vi "Reveal World.vi"(6 "radius":i32 min=0, 8 "y":i32 min=0, 9 "x":i32 min=0, 10 "cost in":dbl[][](array[numeric]), 11 "map reference in":refnum<data-value>) -> (2 "cost out":dbl[][](array[numeric]), 3 "map reference in 2":refnum<data-value>)   [LabVIEW 2013]
uses:
  <vilib>/robotics/Navigation/shared/WorldMap/OccupancyGridWorldMap/NI_Robotics_OccupancyGridWorldMap.lvclass
panel:
  in  "error in (no error)":errorcluster
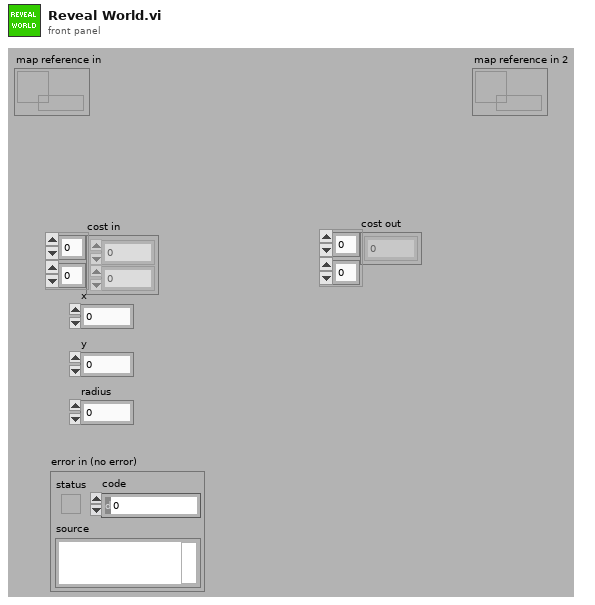
[diagram p1: front panel]
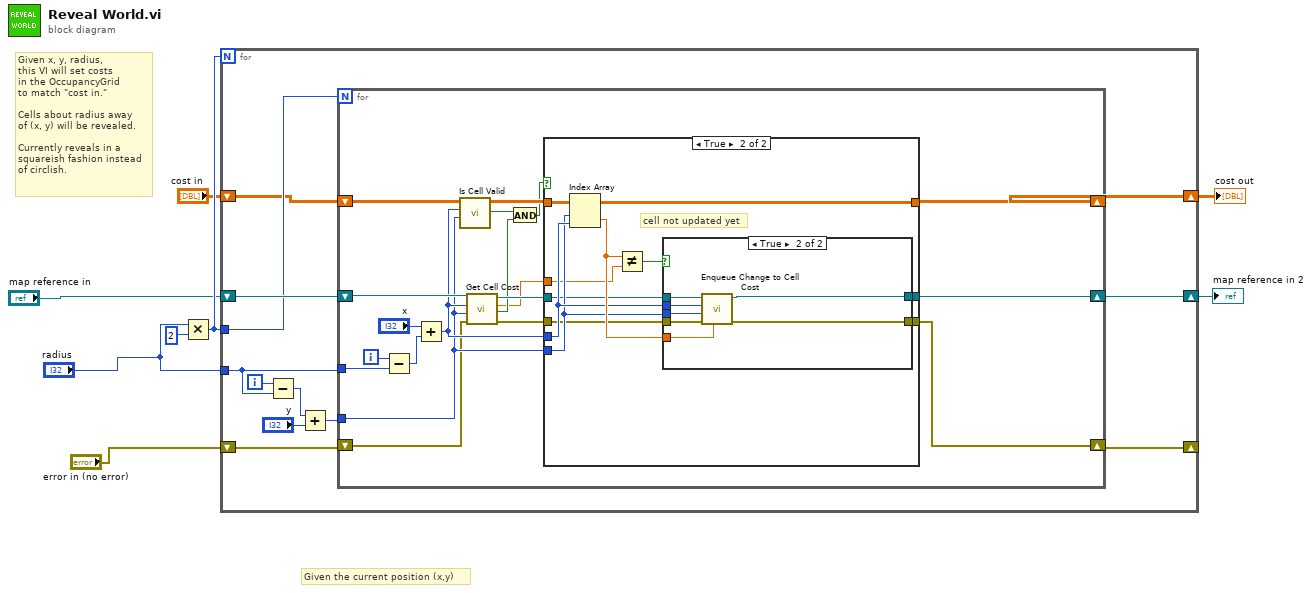
[diagram p0: block diagram]
diagram:
  # "Given the current position (x,y)"
  # "Given x, y, radius,\nthis VI will set costs\nin the OccupancyGrid\nto match \"cost in.\"\n\nCells about radius away\nof (x, y) will be revealed.\n\nCurrently reveals in a \nsquareish fashion instead\nof circlish."
  n1 = Multiply(x="radius", y=2) -> (x*y=w7:i32)
  n2 = for {
    N: w7 -> [_]
    shift-right: [w19] -> w3
    shift-left: "map reference in" -> [w20]
    tunnel: w7 -> [w18]
    tunnel: "radius" -> [w16]
    shift-right: [w14] -> w5
    shift-left: "cost in" -> [w15]
    shift-right: [w9] -> _
    shift-left: "error in (no error)" -> [w10]
    i -> [w17]
    n3 = Subtract(x=w17, y=w16) -> (x-y=w13:i32)
    n4 = Add(x=w13, y="y") -> (x+y=w11:i32)
    n5 = for {
      N: w18 -> [_]
      shift-right: [w21] -> w19
      shift-left: w20 -> [w30]
      tunnel: w16 -> [w38]
      tunnel: w11 -> [w27]
      shift-right: [w35] -> w14
      shift-left: w15 -> [w37]
      shift-right: [w22] -> w9
      shift-left: w10 -> [w24]
      i -> [w39]
      n6 = Subtract(x=w39, y=w38) -> (x-y=w33:i32)
      n7 = Add(x="x", y=w33) -> (x+y=w28:i32)
      n8 = call "Is Cell Valid.vi"("y"=w27, "x"=w28, "cost in"=w37) -> ("Valid"=w31:bool, "cost out"=w36:dbl[][])  [unwired: 7 in]
      n9 = call <vilib>:"Get Cell Cost.vi"("error in (no error)"=w24, "y"=w27, "x"=w28, "map reference in"=w30) -> ("error out"=w23:errorcluster, "found?"=w26:bool, "cost"=w25:dbl, "map reference out"=w29:refnum<data-value>)  [unwired: 4 in]
      n10 = And(x=w31, y=w26) -> (x .and. y?=w34:bool)
      n11 = case shown="True" w34 {
        tunnel: [w42 w52] -> w21
        tunnel: w29 -> [w42 w46]
        tunnel: w28 -> [_ w49]
        tunnel: w27 -> [_ w48]
        tunnel: w36 -> [w41 w43]
        tunnel: [w41 w43] -> w35
        tunnel: w25 -> [_ w47]
        tunnel: w23 -> [w40 w45]
        tunnel: [w40 w44] -> w22
        frame False {
        }
        frame True {
          # "cell not updated yet"
          n12 = Index Array(array=w43, index (row)=w48, index (col)=w49) -> (element=w50:dbl)
          n13 = Not Equal?(x=w50, y=w47) -> (x != y?=w51:bool)
          n14 = case shown="True" w51 {
            tunnel: [w54 w55] -> w52
            tunnel: w46 -> [w54 w61]
            tunnel: w49 -> [_ w60]
            tunnel: w48 -> [_ w59]
            tunnel: w50 -> [_ w58]
            tunnel: w45 -> [w53 w57]
            tunnel: [w53 w56] -> w44
            frame False {
            }
            frame True {
              n15 = call <vilib>:"Enqueue Change to Cell Cost.vi"("cost"=w58, "error in (no error)"=w57, "y"=w59, "x"=w60, "map reference in"=w61) -> ("error out"=w56:errorcluster, "map reference out"=w55:refnum<data-value>)  [unwired: 5 in]
            }
          }
        }
      }
    }
  }
  "cost out" <- w5
  "map reference in 2" <- w3
